vi "Open Swerve Drive.vi"   [LabVIEW 2017]
uses:
  <vilib>/Rock Robotics/WPI/ThirdParty/Phoenix-LabVIEW/Motor Controller/Controls/CTRE_Phoenix_MotorControl_ControlMode.ctl
  <vilib>/Rock Robotics/WPI/ThirdParty/Phoenix-LabVIEW/Motor Controller/Controls/CTRE_Phoenix_MotorControl_FeedbackDevice.ctl
types:
  T1 = enum16{"DemandType_Neutral", "DemandType_AuxPID", "DemandType_ArbitraryFeedForward"}
  T2 = typedef "CTRE_Phoenix_MotorControl_FeedbackDevice.ctl" = i8
  T3 = typedef "CTRE_Phoenix_MotorControl_ControlMode.ctl" = u16
  T4 = typedef "WPI_MotorControlDeviceRef.ctl" = cluster{"DeviceStatus":errorcluster, "Type":T5, "PWM":cluster{"PWM Channel":T6, "DeadBand":T7}, "CAN":cluster{"Device Number":u8, "SetOutput VI Ref":variant, "GetOutput VI Ref":variant, "Enable VI Ref":variant, "Disable VI Ref":variant, "Data":variant}, "Invert":bool, "DIO PWM":cluster{"PWM \"Enable\" Channel":T6, "DIOChannel":T8, "PWM Rate":dbl}}
  T5 = typedef "WPI_MotorControlType.ctl" = enum16{"PWM", "CAN", "DIO PWM"}
  T6 = typedef "FPGA_DIOPWMChannel.ctl" = enum8{"PWM 0", "PWM 1", "PWM 2", "PWM 3", "PWM 4", "PWM 5", "PWM 6", "PWM 7", "PWM 8", "PWM 9", "PWM MXP 0", "PWM MXP 1", "PWM MXP 2", "PWM MXP 3", "PWM MXP 4", "PWM MXP 5", "PWM MXP 6", "PWM MXP 7", "PWM MXP 8", "PWM MXP 9", "Invalid"}
  T7 = typedef "WPI_PWMDeadband.ctl" = cluster{"Name":string, "maxPositivePwm":i32, "minPositivePwm":i32, "centerPwm":i32, "maxNegativePwm":i32, "minNegativePwm":i32, "angularRange":u16}
  T8 = typedef "FPGA_DIOChannel.ctl" = enum8{"DIO 0", "DIO 1", "DIO 2", "DIO 3", "DIO 4", "DIO 5", "DIO 6", "DIO 7", "DIO 8", "DIO 9", "DIO MXP 0", "DIO MXP 1", "DIO MXP 2", "DIO MXP 3", "DIO MXP 4", "DIO MXP 5", "DIO MXP 6", "DIO MXP 7", "DIO MXP 8", "DIO MXP 9", "DIO MXP 10", "DIO MXP 11", "DIO MXP 12", "DIO MXP 13", "DIO MXP 14", "DIO MXP 15", "SPI Port CS1", "SPI Port CS2", "SPI Port CS3", "SPI Port MISO", "SPI Port MOSI", "Invalid"}
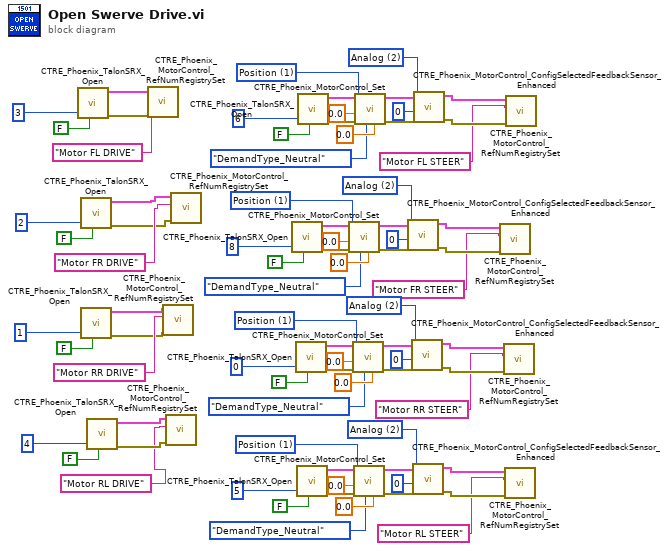
[diagram p0: block diagram]
diagram:
  w8 = T2 2 items=["None"=-1, "QuadEncoder"=0, "Analog"=2, "Tachometer"=4, "Pulse Width Encoded Position"=8, "Sensor Sum (S0 + S1)"=9, "Sensor Difference (D0 - D1)"=10, "Remote Source 0"=11, "Remote Source 1"=12, "Software Emulated"=15] ("Feedback Device")
  w11 = T3 1 items=["PercentOutput"=0, "Position"=1, "Velocity"=2, "Current"=3, "Follower"=5, "MotionProfile"=6, "MotionMagic"=7, "MotionMagicArc"=8, "MotionProfileArc"=10, "Disabled"=15] ("Control Mode")
  w23 = T2 2 items=["None"=-1, "QuadEncoder"=0, "Analog"=2, "Tachometer"=4, "Pulse Width Encoded Position"=8, "Sensor Sum (S0 + S1)"=9, "Sensor Difference (D0 - D1)"=10, "Remote Source 0"=11, "Remote Source 1"=12, "Software Emulated"=15] ("Feedback Device")
  w26 = T3 1 items=["PercentOutput"=0, "Position"=1, "Velocity"=2, "Current"=3, "Follower"=5, "MotionProfile"=6, "MotionMagic"=7, "MotionMagicArc"=8, "MotionProfileArc"=10, "Disabled"=15] ("Control Mode")
  w38 = T2 2 items=["None"=-1, "QuadEncoder"=0, "Analog"=2, "Tachometer"=4, "Pulse Width Encoded Position"=8, "Sensor Sum (S0 + S1)"=9, "Sensor Difference (D0 - D1)"=10, "Remote Source 0"=11, "Remote Source 1"=12, "Software Emulated"=15] ("Feedback Device")
  w41 = T3 1 items=["PercentOutput"=0, "Position"=1, "Velocity"=2, "Current"=3, "Follower"=5, "MotionProfile"=6, "MotionMagic"=7, "MotionMagicArc"=8, "MotionProfileArc"=10, "Disabled"=15] ("Control Mode")
  w53 = T2 2 items=["None"=-1, "QuadEncoder"=0, "Analog"=2, "Tachometer"=4, "Pulse Width Encoded Position"=8, "Sensor Sum (S0 + S1)"=9, "Sensor Difference (D0 - D1)"=10, "Remote Source 0"=11, "Remote Source 1"=12, "Software Emulated"=15] ("Feedback Device")
  w56 = T3 1 items=["PercentOutput"=0, "Position"=1, "Velocity"=2, "Current"=3, "Follower"=5, "MotionProfile"=6, "MotionMagic"=7, "MotionMagicArc"=8, "MotionProfileArc"=10, "Disabled"=15] ("Control Mode")
  n1 = call <vilib>:"CTRE_Phoenix_TalonSRX_Open.vi"("Invert"=FALSE, "Device Number"=u8 3) -> ("error out"=w76:errorcluster, "CAN Talon SRX Ref"=w77:T4)  [unwired: 8 in]
  n2 = call <vilib>:"CTRE_Phoenix_TalonSRX_Open.vi"("Invert"=FALSE, "Device Number"=u8 2) -> ("error out"=w63:errorcluster, "CAN Talon SRX Ref"=w65:T4)  [unwired: 8 in]
  n3 = call <vilib>:"CTRE_Phoenix_TalonSRX_Open.vi"("Invert"=FALSE, "Device Number"=u8 1) -> ("error out"=w60:errorcluster, "CAN Talon SRX Ref"=w62:T4)  [unwired: 8 in]
  n4 = call <vilib>:"CTRE_Phoenix_TalonSRX_Open.vi"("Invert"=FALSE, "Device Number"=u8 4) -> ("error out"=w58:errorcluster, "CAN Talon SRX Ref"=w59:T4)  [unwired: 8 in]
  n5 = call <vilib>:"CTRE_Phoenix_MotorControl_RefNumRegistrySet.vi"("error in (no error)"=w76, "refnum name"="Motor FL DRIVE", "PhoenixMotorControlDevRef"=w77) -> ()  [unwired: 7 in, 2 out]
  n6 = call <vilib>:"CTRE_Phoenix_MotorControl_RefNumRegistrySet.vi"("error in (no error)"=w60, "refnum name"="Motor RR DRIVE", "PhoenixMotorControlDevRef"=w62) -> ()  [unwired: 7 in, 2 out]
  n7 = call <vilib>:"CTRE_Phoenix_MotorControl_RefNumRegistrySet.vi"("error in (no error)"=w58, "refnum name"="Motor RL DRIVE", "PhoenixMotorControlDevRef"=w59) -> ()  [unwired: 7 in, 2 out]
  n8 = call <vilib>:"CTRE_Phoenix_MotorControl_RefNumRegistrySet.vi"("error in (no error)"=w63, "refnum name"="Motor FR DRIVE", "PhoenixMotorControlDevRef"=w65) -> ()  [unwired: 7 in, 2 out]
  n9 = call <vilib>:"CTRE_Phoenix_TalonSRX_Open.vi"("Invert"=FALSE, "Device Number"=u8 8) -> ("error out"=w42:errorcluster, "CAN Talon SRX Ref"=w43:T4)  [unwired: 8 in]
  n10 = call <vilib>:"CTRE_Phoenix_TalonSRX_Open.vi"("Invert"=FALSE, "Device Number"=u8 0) -> ("error out"=w27:errorcluster, "CAN Talon SRX Ref"=w28:T4)  [unwired: 8 in]
  n11 = call <vilib>:"CTRE_Phoenix_TalonSRX_Open.vi"("Invert"=FALSE, "Device Number"=u8 5) -> ("error out"=w12:errorcluster, "CAN Talon SRX Ref"=w13:T4)  [unwired: 8 in]
  n12 = call <vilib>:"CTRE_Phoenix_TalonSRX_Open.vi"("Invert"=FALSE, "Device Number"=u8 6) -> ("error out"=w66:errorcluster, "CAN Talon SRX Ref"=w67:T4)  [unwired: 8 in]
  n13 = call <vilib>:"CTRE_Phoenix_MotorControl_Set.vi"("Demand1"=0.0, "DemandType"=T1."DemandType_Neutral", "error in (no error)"=w42, "Output"=0.0, "Control Mode"=w41, "PhoenixMotorControlDevRef"=w43) -> ("error out"=w40:errorcluster, "PhoenixMotorControlDevRef"=w39:T4)  [unwired: 4 in]
  n14 = call <vilib>:"CTRE_Phoenix_MotorControl_Set.vi"("Demand1"=0.0, "DemandType"=T1."DemandType_Neutral", "error in (no error)"=w27, "Output"=0.0, "Control Mode"=w26, "PhoenixMotorControlDevRef"=w28) -> ("error out"=w25:errorcluster, "PhoenixMotorControlDevRef"=w24:T4)  [unwired: 4 in]
  n15 = call <vilib>:"CTRE_Phoenix_MotorControl_Set.vi"("Demand1"=0.0, "DemandType"=T1."DemandType_Neutral", "error in (no error)"=w12, "Output"=0.0, "Control Mode"=w11, "PhoenixMotorControlDevRef"=w13) -> ("error out"=w10:errorcluster, "PhoenixMotorControlDevRef"=w9:T4)  [unwired: 4 in]
  n16 = call <vilib>:"CTRE_Phoenix_MotorControl_Set.vi"("Demand1"=0.0, "DemandType"=T1."DemandType_Neutral", "error in (no error)"=w66, "Output"=0.0, "Control Mode"=w56, "PhoenixMotorControlDevRef"=w67) -> ("error out"=w55:errorcluster, "PhoenixMotorControlDevRef"=w54:T4)  [unwired: 4 in]
  n17 = call <vilib>:"CTRE_Phoenix_MotorControl_ConfigSelectedFeedbackSensor_Enhanced.vi"("error in (no error)"=w40, "pidLoopIdx"=0, "Feedback Device"=w38, "PhoenixMotorControlDevRef"=w39) -> ("error out"=w36:errorcluster, "PhoenixMotorControlDevRef"=w37:T4)  [unwired: 6 in]
  n18 = call <vilib>:"CTRE_Phoenix_MotorControl_ConfigSelectedFeedbackSensor_Enhanced.vi"("error in (no error)"=w25, "pidLoopIdx"=0, "Feedback Device"=w23, "PhoenixMotorControlDevRef"=w24) -> ("error out"=w21:errorcluster, "PhoenixMotorControlDevRef"=w22:T4)  [unwired: 6 in]
  n19 = call <vilib>:"CTRE_Phoenix_MotorControl_ConfigSelectedFeedbackSensor_Enhanced.vi"("error in (no error)"=w10, "pidLoopIdx"=0, "Feedback Device"=w8, "PhoenixMotorControlDevRef"=w9) -> ("error out"=w6:errorcluster, "PhoenixMotorControlDevRef"=w7:T4)  [unwired: 6 in]
  n20 = call <vilib>:"CTRE_Phoenix_MotorControl_ConfigSelectedFeedbackSensor_Enhanced.vi"("error in (no error)"=w55, "pidLoopIdx"=0, "Feedback Device"=w53, "PhoenixMotorControlDevRef"=w54) -> ("error out"=w51:errorcluster, "PhoenixMotorControlDevRef"=w52:T4)  [unwired: 6 in]
  n21 = call <vilib>:"CTRE_Phoenix_MotorControl_RefNumRegistrySet.vi"("error in (no error)"=w36, "refnum name"="Motor FR STEER", "PhoenixMotorControlDevRef"=w37) -> ()  [unwired: 7 in, 2 out]
  n22 = call <vilib>:"CTRE_Phoenix_MotorControl_RefNumRegistrySet.vi"("error in (no error)"=w21, "refnum name"="Motor RR STEER", "PhoenixMotorControlDevRef"=w22) -> ()  [unwired: 7 in, 2 out]
  n23 = call <vilib>:"CTRE_Phoenix_MotorControl_RefNumRegistrySet.vi"("error in (no error)"=w6, "refnum name"="Motor RL STEER", "PhoenixMotorControlDevRef"=w7) -> ()  [unwired: 7 in, 2 out]
  n24 = call <vilib>:"CTRE_Phoenix_MotorControl_RefNumRegistrySet.vi"("error in (no error)"=w51, "refnum name"="Motor FL STEER", "PhoenixMotorControlDevRef"=w52) -> ()  [unwired: 7 in, 2 out]
